vi "FG_FPGA_Interface_WPC.vi"(5 "Invert Dir?":bool, 7 "Action":T1, 8 "error in":errorcluster) -> (0 "error out":errorcluster, 3 "FPGA VI Reference Out":refnum<k20>)   [LabVIEW 2015]
uses:
  Typedef_FPGA_Interface_Action.ctl
  <vilib>/FPGAPlugInAG/sbRIO-9606/niLvFpga_Open_sbRIO-9606.vi
  <vilib>/rvi/interface/common/dynamic/niFpgaDynamicAddResources.vi
  <vilib>/Utility/error.llb/Error Cluster From Error Code.vi
  <vilib>/rvi/errors/niLvFpgaAdjustHostInterfaceError.vi
  <vilib>/nisyscfg/Initialize (Control).vi
  <vilib>/nisyscfg/Find Hardware.vi
  <vilib>/FPGAPlugInAG/Dynamic/niLvFpga_Close_Dynamic.vi
  <vilib>/rvi/interface/nirviOpenFPGA/nirviOpenFPGA.xnode
  FPGA Bitfiles/Main FPGA 8-axis for WPC.lvbitx
  <vilib>/rvi/interface/nirviReadWriteControl/nirviReadWriteControl.xnode
  <vilib>/rvi/interface/nirviCloseFPGA/nirviCloseFPGA.xnode
  <vilib>/nisyscfg/nisyscfg.lvlib
  <vilib>/rvi/interface/Simulation/niFpgaSimulationCallBeginRW.vi
  NiFpgaLv.dll
panel:
  out "Numeric":i32
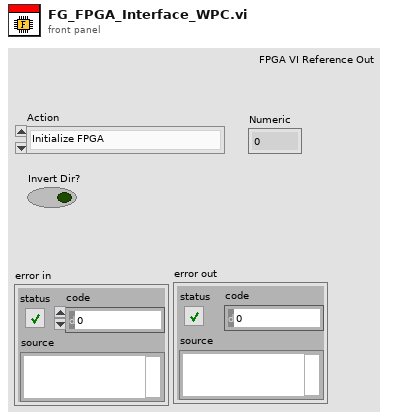
[diagram p1: front panel]
types:
  T1 = typedef "Typedef_FPGA_Interface_Action.ctl" = enum16{"Initialize FPGA", "Get FPGA Reference", "Close FPGA"}
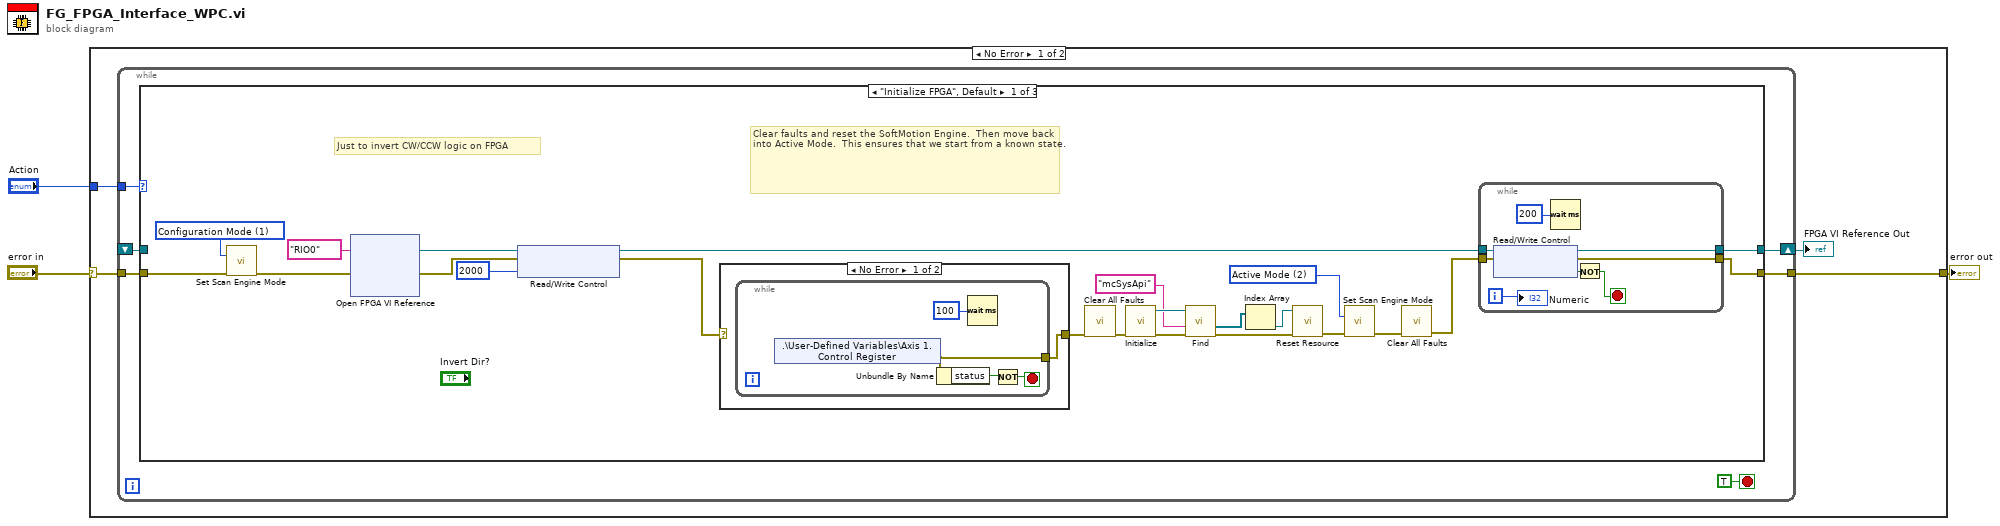
[diagram p0: block diagram]
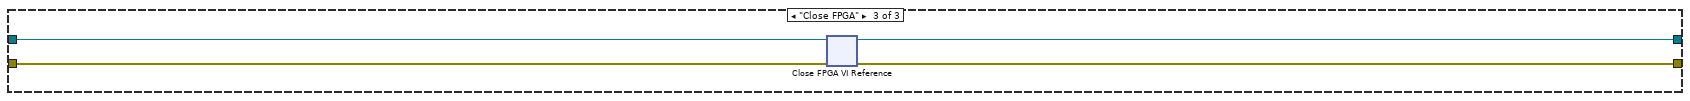
[diagram p4: hidden frame]
diagram:
  n1 = case shown="No Error" "error in" {
    selector: "error in" -> [w7 w56]
    tunnel: [w6 w56] -> w2
    tunnel: "Action" -> [w5 _]
    frame No Error {
      n2 = while {
        tunnel: w7 -> [w11]
        tunnel: w5 -> [w12]
        tunnel: [w10] -> w6
        shift-right: [w9] -> w4
        shift-left: _ -> [w8]
        stop <- TRUE stop-if-true
        n3 = case shown="\"Initialize FPGA\", Default" w12 {
          tunnel: w11 -> [w35 w51 w54]
          tunnel: [w19 w51 w55] -> w10
          tunnel: w8 -> [_ w52 w53]
          tunnel: [w20 w52 w53] -> w9
          frame "Initialize FPGA", Default {
            w22 = 2 items=["Configuration Mode"=1, "Active Mode"=2] ("mode (Active Mode)")
            w30 = 1 items=["Configuration Mode"=1, "Active Mode"=2] ("mode (Active Mode)")
            # "Just to invert CW/CCW logic on FPGA"
            # "Clear faults and reset the SoftMotion Engine.  Then move back into Active Mode.  This ensures that we start from a known state."
            n4 = call <vilib>:"Set Scan Engine Mode.vi"("mode (Active Mode)"=w30, "error in (no error)"=w35) -> ("error out"=w34:errorcluster)  [unwired: 13 in]
            n5 = xnode "Open FPGA VI Reference"("error in"=w34, "resource name"=tag "RIO0") -> ("FPGA VI Reference Out"=w17:refnum<k20>, "error out"=w18:errorcluster)
            n6 = xnode "Read/Write Control"("FPGA VI Reference In"=w17, "error in"=w18, "minimum pulse"=u16 2000) -> ("FPGA VI Reference Out"=w21:refnum<k20>, "error out"=w32:errorcluster)
            n7 = case shown="No Error" w32 {
              selector: w32 -> [_ w50]
              tunnel: [w45 w50] -> w33
              frame No Error {
                n8 = while {
                  tunnel: [w46] -> w45
                  stop <- w49 stop-if-true
                  n9 = shared-variable ".\\User-Defined Variables\\Axis 1.Control Register"() -> (error out=w46:errorcluster)  [unwired: 1 in, 1 out]
                  n10 = Unbundle By Name(w46) -> ("status"=w48:bool)
                  n11 = Wait (ms)(milliseconds to wait=u32 100) -> ()  [unwired: 1 out]
                  n12 = Not(x=w48) -> (.not. x?=w49:bool)
                }
              }
              frame Error {
              }
            }
            n13 = call <vilib>:"Clear All Faults.vi"("error in (no error)"=w33) -> ("error out"=w29:errorcluster)  [unwired: 10 in]
            n14 = call-poly <vilib>:"Initialize.vi"("error in (no error)"=w29) -> ("error out"=w23:errorcluster, "Session out"=w25:refnum<k21>)  [unwired: 8 in, 1 out]
            n15 = call-poly <vilib>:"Find.vi"("error in (no error)"=w23, "Experts"="mcSysApi" ("experts"), "Session in"=w25) -> ("error out"=w28:errorcluster, "Resources out"=w26:refnum<k20>[])  [unwired: 5 in, 2 out]
            n16 = Index Array(array=w26) -> (element=w27:refnum<k20>)  [unwired: 1 in]
            n17 = call <vilib>:"Reset Resource.vi"("error in (no error)"=w28, "Resource in"=w27) -> ("error out"=w16:errorcluster)  [unwired: 6 in, 3 out]
            n18 = call <vilib>:"Set Scan Engine Mode.vi"("mode (Active Mode)"=w22, "error in (no error)"=w16) -> ("error out"=w15:errorcluster)  [unwired: 13 in]
            n19 = call <vilib>:"Clear All Faults.vi"("error in (no error)"=w15) -> ("error out"=w14:errorcluster)  [unwired: 10 in]
            n20 = while {
              tunnel: w14 -> [w44]
              tunnel: [w43] -> w19
              tunnel: w21 -> [w39]
              tunnel: [w38] -> w20
              i -> [w37]
              stop <- w40 stop-if-true
              n21 = xnode "Read/Write Control"("FPGA VI Reference In"=w39, "error in"=w44) -> ("FPGA VI Reference Out"=w38:refnum<k20>, "error out"=w43:errorcluster, "Sync is Fault"=w42:bool)
              n22 = Wait (ms)(milliseconds to wait=u32 200) -> ()  [unwired: 1 out]
              n23 = Not(x=w42) -> (.not. x?=w40:bool)
              "Numeric" <- w37
            }
          }
          frame "Get FPGA Reference" {
          }
          frame "Close FPGA" {
            n24 = xnode "Close FPGA VI Reference"("FPGA VI Reference In"=w53, "error in"=w54) -> ("error out"=w55:errorcluster)
          }
        }
      }
      "FPGA VI Reference Out" <- w4
    }
    frame Error {
    }
  }
  "error out" <- w2
